vi "Real Time Clock (DS1307) - SET-GET Date Time.vi"() -> ()   [LabVIEW 2014]
doc: "This example shows how to set and get date/time from DS1307 RTC IC. To set the current time, enable the \"Set\" control and populate the date structure with the current date/time, then download the code first. Then turn off \"Set\" and download again to read the time only. The current date/time will be maintained after power cycle if the battery is installed in the shield."
uses:
  QwaveSys_Interface/QwaveSys_Interface.lvlib
  PWS_ESP8266/PWS_ESP8266.lvlib
panel:
  in  "Set Date/Time":bool
  in  "time string":string="01:15:00"
  in  "date string":string="Jan 04 2015"
  # "Overview: Demonstrates how to set and read the date/time of DS1307 RTC IC. To set the current time, enable the \"Set\" control and populate the date structure with the current date/time, then download the code first.  Then turn off \"Set\" and download again to read the time only.  The current date/time will be maintained after power cycle if the battery is installed in the module.\nRequirements: LabVIEW Full Development System,Arduino Compatible Compiler for LabVIEW,Programmable Wireless Stamp (PWS) Library.\nInstructions:\n1. Insert CR20xx 3V RTC backup battery.\n2. Enable \"Set\" and set the current date/time.\n3.  Open Tools>Arduino Compatible Compiler for LabVIEW in LabVIEW, then select File>Load VI, and select this VI and then Compile and Download.\n4. Then disable \"Set\" and Compile and Download again.\n5. Open a serial terminal and observe the current date and time being printed."
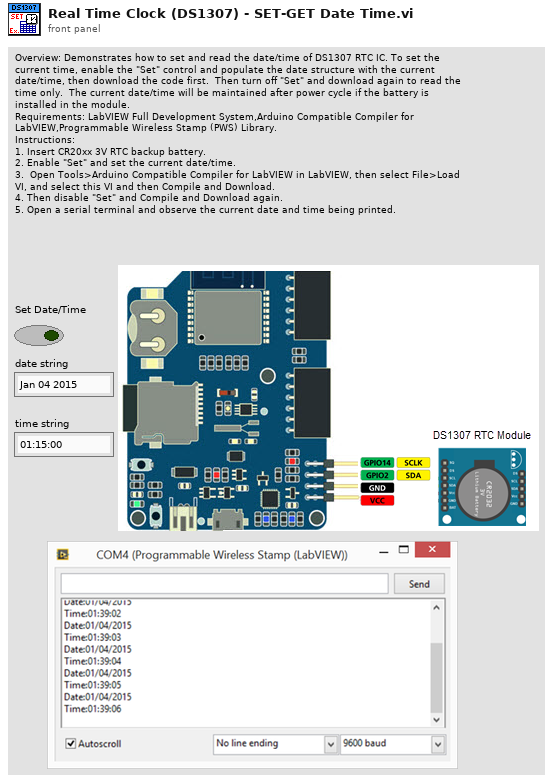
[diagram p1: front panel]
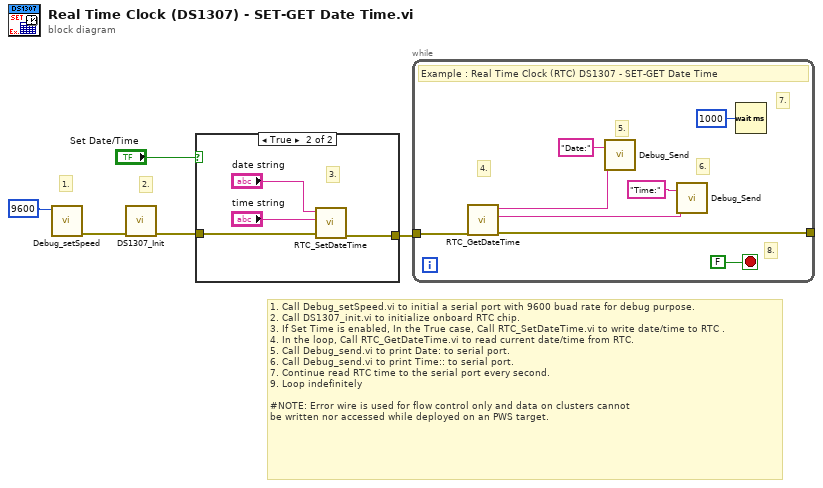
[diagram p0: block diagram]
diagram:
  # "2."
  # "1."
  # "1. Call Debug_setSpeed.vi to initial a serial port with 9600 buad rate for debug purpose.\n2. Call DS1307_init.vi to initialize onboard RTC chip.\n3. If Set Time is enabled, In the True case, Call RTC_SetDateTime.vi to write date/time to RTC .\n4. In the loop, Call RTC_GetDateTime.vi to read current date/time from RTC.\n5. Call Debug_send.vi to print Date: to serial port. \n6. Call Debug_send.vi to print Time:: to serial port. \n7. Continue read RTC time to the serial port every second.\n9. Loop indefinitely\n\n#NOTE: Error wire is used for flow control only and data on clusters cannot\nbe written nor accessed while deployed on an PWS target."
  n1 = call "Debug_setSpeed.vi"("Speed"=u32 9600) -> ("error out"=w2:errorcluster)  [unwired: 10 in]
  n2 = call "DS1307_Init.vi"("error in (no error)"=w2) -> ("error out"=w1:errorcluster)  [unwired: 10 in]
  n3 = case shown="True" "Set Date/Time" {
    tunnel: [w6 w10] -> w4
    tunnel: w1 -> [w6 w9]
    frame False {
    }
    frame True {
      # "3."
      n4 = call "RTC_SetDateTime.vi"("error in (no error)"=w9, "time string"="time string", "date string"="date string") -> ("error out"=w10:errorcluster)  [unwired: 8 in]
    }
  }
  n5 = while {
    tunnel: w4 -> [w18]
    tunnel: [w13] -> _
    stop <- FALSE stop-if-true
    # "8."
    # "7."
    # "6."
    # "5."
    # "4."
    # "Example : Real Time Clock (RTC) DS1307 - SET-GET Date Time"
    n6 = call "RTC_GetDateTime.vi"("error in (no error)"=w18) -> ("error out"=w13:errorcluster, "time string"=w15:string, "date string"=w16:string)  [unwired: 8 in]
    n7 = call "Debug_Send.vi"("Name"="Date:", "DATA"=w16) -> ()  [unwired: 10 in]
    n8 = call "Debug_Send.vi"("Name"="Time:", "DATA"=w15) -> ()  [unwired: 10 in]
    n9 = Wait (ms)(milliseconds to wait=u32 1000) -> ()  [unwired: 1 out]
  }
